vi "Agilent_Error Query.vi"(8 "error in (no error)":errorcluster, 11 "VISA resource name":refnum<visa-resource-name>) -> (0 "error out":errorcluster, 1 "Error Message":string, 2 "Error Code":i32[](array[numeric]), 3 "VISA resource name out":refnum<visa-resource-name>)   [LabVIEW 2020]
doc: "This VI queries the instrument for any errors in the instrument's error queue. It will continue to read errors until all errors have been read from the instrument. Any errors will be returned in the Error Out cluster.\n\n<B>Note:</B>\n\nThis VI is called automatically by most driver VIs so it is not usually necessary to call this in an application."
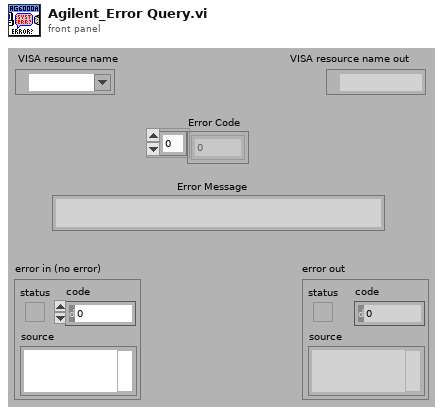
[diagram p1: front panel]
types:
  T1 = cluster{"show call chain? (False)":bool, "Code":i32, string}
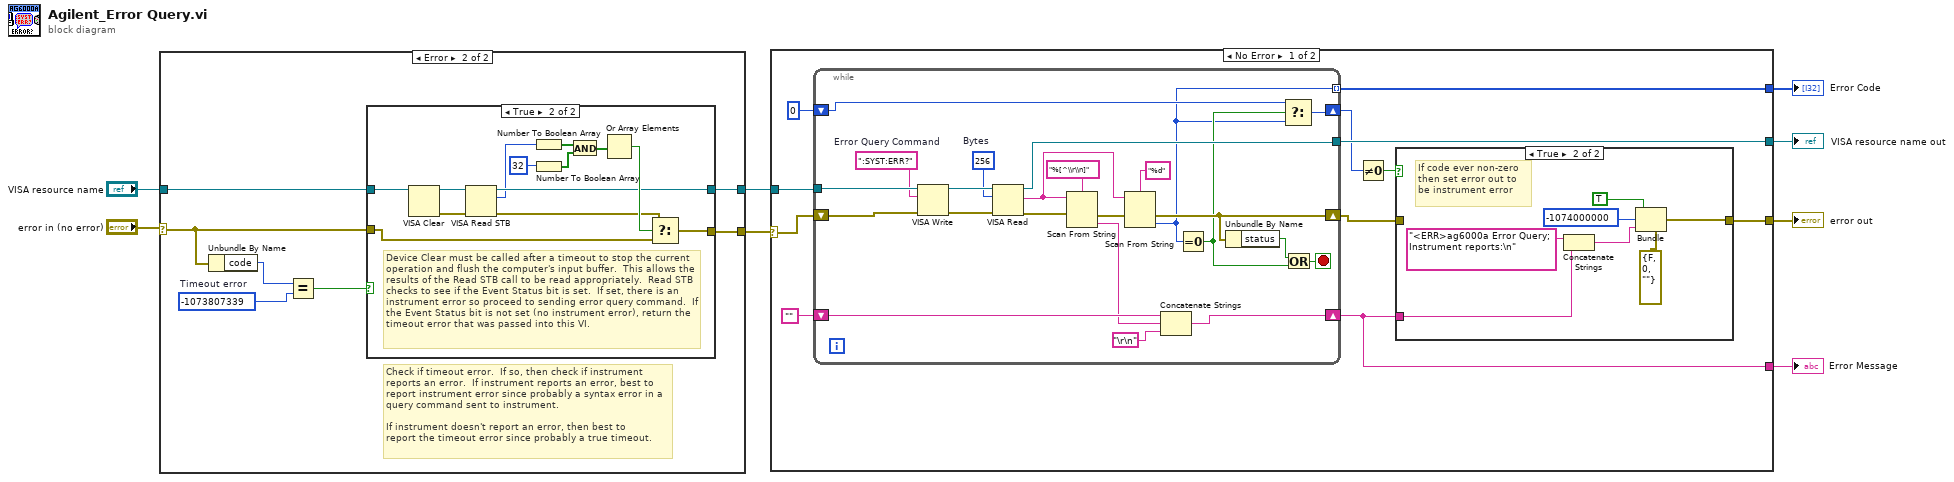
[diagram p0: block diagram]
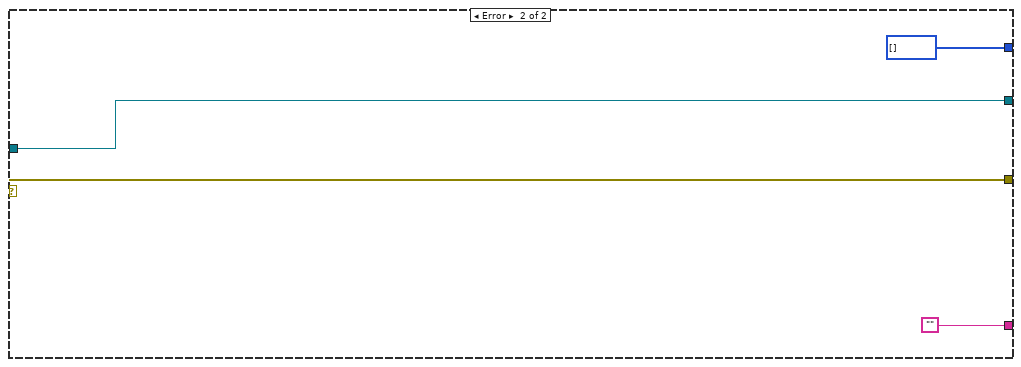
[diagram p5: hidden frame]
diagram:
  n1 = case shown="Error" "error in (no error)" {
    selector: "error in (no error)" -> [w9 w14]
    tunnel: "VISA resource name" -> [w10 w17]
    tunnel: [w10 w15] -> w3
    tunnel: [w9 w13] -> w1
    frame No Error {
    }
    frame Error {
      w16 = -1073807339  # Timeout error
      # "Check if timeout error.  If so, then check if instrument reports an error.  If instrument reports an error, best to report instrument error since probably a syntax error in a query command sent to instrument.\n\nIf instrument doesn't report an error, then best to \nreport the timeout error since probably a true timeout."
      n2 = Unbundle By Name(w14) -> ("code"=w12:i32)
      n3 = Equal?(x=w12, y=w16) -> (x = y?=w11:bool)
      n4 = case shown="True" w11 {
        tunnel: w17 -> [w19 w25]
        tunnel: [w19 w21] -> w15
        tunnel: w14 -> [w18 w28]
        tunnel: [w18 w27] -> w13
        frame False {
          # "Error code not a timeout, so best to pass on to user."
        }
        frame True {
          # "Device Clear must be called after a timeout to stop the current operation and flush the computer's input buffer.  This allows the results of the Read STB call to be read appropriately.  Read STB checks to see if the Event Status bit is set.  If set, there is an instrument error so proceed to sending error query command.  If the Event Status bit is not set (no instrument error), return the timeout error that was passed into this VI."
          n5 = VISA Clear(VISA resource name=w25) -> (VISA resource name out=w24:refnum<visa-resource-name>, error out=w23:errorcluster)  [unwired: 1 in]
          n6 = VISA Read STB(8:w23, 11:w24) -> (0:w22:errorcluster, 2:w20:u16, 3:w21:refnum<visa-resource-name>)
          n7 = Number To Boolean Array(number=w20) -> (Boolean array=w29:bool[])
          n8 = Number To Boolean Array(number=32) -> (Boolean array=w31:bool[])
          n9 = And(x=w29, y=w31) -> (x .and. y?=w30:bool[])
          n10 = Or Array Elements(Boolean array=w30) -> (logical OR=w26:bool)
          n11 = Select(t=w22, s=w26, f=w28) -> (s? t:f=w27:errorcluster)
        }
      }
    }
  }
  n12 = case shown="No Error" w1 {
    selector: w1 -> [w35 w75]
    tunnel: [w43 w78] -> w8
    tunnel: w3 -> [w34 w78]
    tunnel: [w36 w75] -> w6
    tunnel: [w37 "" ("Empty String Constant")] -> w5
    tunnel: [w39 i32[] []] -> w4
    frame No Error {
      n13 = while {
        tunnel: [w74] -> w43
        tunnel: w34 -> [w73]
        shift-right: [w61] -> w37
        shift-left: "" ("Empty String Constant") -> [w64]
        shift-right: [w59] -> w40
        shift-left: 0 -> [w60]
        shift-right: [w57] -> w33
        shift-left: w35 -> [w58]
        tunnel: [w52] -> w39 mode=indexing
        stop <- w67 stop-if-true
        w71 = u32 256  # Bytes
        w69 = ":SYST:ERR?"  # Error Query Command
        n14 = VISA Write(VISA resource name=w73, write buffer=w69, error in (no error)=w58) -> (VISA resource name out=w72:refnum<visa-resource-name>, error out=w70:errorcluster)  [unwired: 1 out]
        n15 = VISA Read(VISA resource name=w72, byte count=w71, error in (no error)=w70) -> (VISA resource name out=w74:refnum<visa-resource-name>, read buffer=w65:string, error out=w56:errorcluster)  [unwired: 1 out]
        n16 = Scan From String(format string="%[^\\r\\n]", input string=w65, error in=w56) -> (error out=w55:errorcluster, output 1=w62:string)  [unwired: 2 in, 2 out]
        n17 = Scan From String(format string="%d", input string=w65, error in=w55) -> (error out=w57:errorcluster, output 1=w52:i32)  [unwired: 2 in, 2 out]
        n18 = Concatenate Strings(w64, w62, "\r\n" ("End of Line Constant")) -> (w61:string)
        n19 = Equal To 0?(x=w52) -> (x = 0?=w53:bool)
        n20 = Unbundle By Name(w57) -> ("status"=w54:bool)
        n21 = Select(t=w60, s=w53, f=w52) -> (s? t:f=w59:i32)
        n22 = Or(x=w54, y=w53) -> (x .or. y?=w67:bool)
      }
      n23 = Not Equal To 0?(x=w40) -> (x != 0?=w38:bool)
      n24 = case shown="True" w38 {
        tunnel: w37 -> [_ w50]
        tunnel: [w44 w45] -> w36
        tunnel: w33 -> [w44 _]
        frame False {
        }
        frame True {
          # "If code ever non-zero\nthen set error out to\nbe instrument error"
          n25 = Concatenate Strings("<ERR>ag6000a Error Query; Instrument reports:\n" ("Source"), w50) -> (w47:string)
          n26 = Bundle(cluster=T1 {"show call chain? (False)"=FALSE, "Code"=0, ""}, "show call chain? (False)"=TRUE, "Code"=-1074000000, w47) -> (w45:T1)
        }
      }
    }
    frame Error {
    }
  }
  "VISA resource name out" <- w8
  "error out" <- w6
  "Error Message" <- w5
  "Error Code" <- w4
